vi "Signal Tracker.vi"(7 "Action":T2, 8 "error in":errorcluster, 11 "Signals":T1[](array[typedef])) -> (0 "error out":errorcluster, 2 "Signal Values":dbl[](array[numeric]), 3 "Signals out":T1[](array[typedef]))   [LabVIEW 2021]
uses:
  controls/Signal Tracker.ctl
  controls/Signal Data.ctl
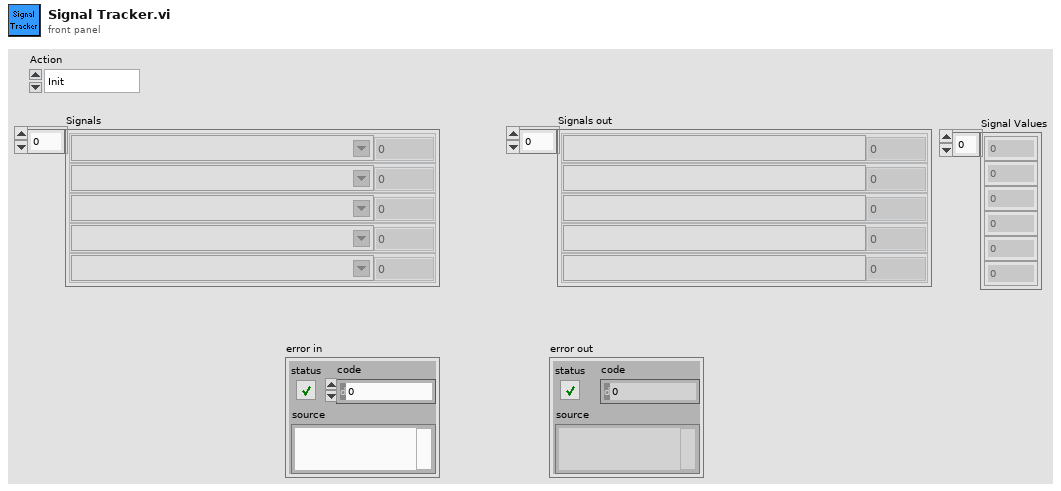
[diagram p1: front panel]
types:
  T1 = typedef "Signal Data.ctl" = cluster{"XNET Signal":refnum<k21>, "Data":dbl}
  T2 = typedef "Signal Tracker.ctl" = enum16{"Init", "Update", "Read", "Clear"}
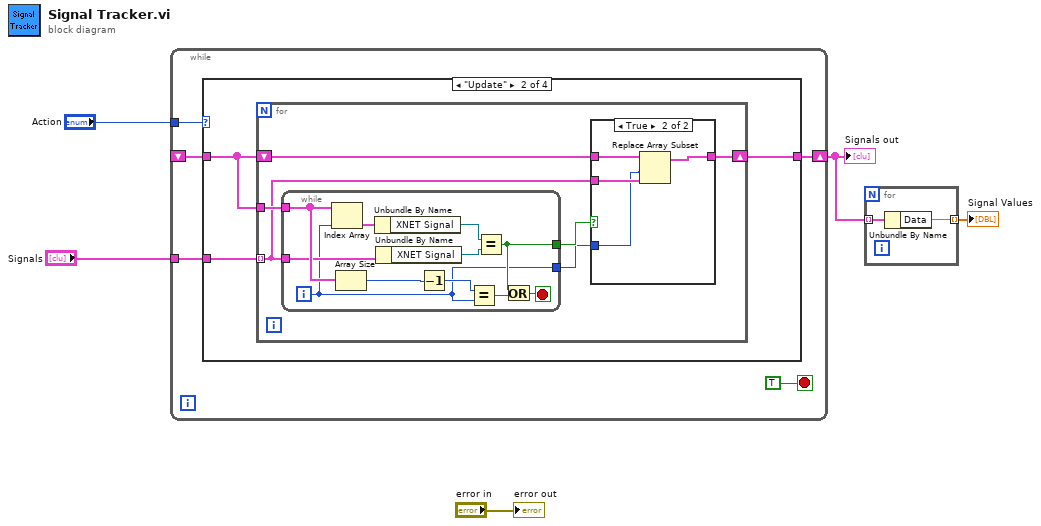
[diagram p0: block diagram]
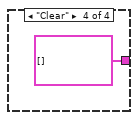
[diagram p5: hidden frame]
diagram:
  n1 = while {
    tunnel: "Action" -> [w9]
    shift-right: [w8] -> w2
    shift-left: _ -> [w7]
    tunnel: "Signals" -> [w6]
    stop <- TRUE stop-if-true
    n2 = case shown="\"Update\"" w9 {
      tunnel: w7 -> [_ w12 w37 _]
      tunnel: [w11 w13 w37 T1[] [] ("Signals")] -> w8
      tunnel: w6 -> [w11 w14 _ _]
      frame "Init" {
      }
      frame "Update" {
        n3 = for {
          tunnel: w14 -> [w17] mode=indexing
          tunnel: w12 -> [w20]
          shift-right: [w16] -> w13
          shift-left: w12 -> [w15]
          n4 = while {
            tunnel: w20 -> [w36]
            tunnel: w17 -> [w30]
            tunnel: [w28] -> w19
            tunnel: [w27] -> w18
            i -> [w27]
            stop <- w26 stop-if-true
            n5 = Index Array(array=w36, index=w27) -> (element=w32:T1)
            n6 = Array Size(array=w36) -> (size(s)=w35:i32)
            n7 = Unbundle By Name(w32) -> ("XNET Signal"=w31:refnum<k21>)
            n8 = Unbundle By Name(w30) -> ("XNET Signal"=w29:refnum<k21>)
            n9 = Decrement(x=w35) -> (x-1=w33:i32)
            n10 = Equal?(x=w33, y=w27) -> (x = y?=w34:bool)
            n11 = Equal?(x=w31, y=w29) -> (x = y?=w28:bool)
            n12 = Or(x=w28, y=w34) -> (x .or. y?=w26:bool)
          }
          n13 = case shown="True" w19 {
            tunnel: w15 -> [w21 w25]
            tunnel: w18 -> [_ w23]
            tunnel: w17 -> [_ w24]
            tunnel: [w21 w22] -> w16
            frame False {
            }
            frame True {
              n14 = Replace Array Subset(array=w25, new element=w24, index=w23) -> (w22:T1[])
            }
          }
        }
      }
      frame "Read" {
      }
      frame "Clear" {
      }
    }
  }
  "Signals out" <- w2
  n15 = for {
    tunnel: w2 -> [w40] mode=indexing
    tunnel: [w39] -> w1 mode=indexing
    n16 = Unbundle By Name(w40) -> ("Data"=w39:dbl)
  }
  "Signal Values" <- w1
  "error out" <- "error in"
